vi "Relabel Annotation.vi"(0 "FSM.Graph In":refnum<class "FSM.Graph.lvclass">, 7 "Old Name":string, 9 "New Name":string) -> (4 "FSM.Graph Out":refnum<class "FSM.Graph.lvclass">)   [LabVIEW 2020, in "FSM.Graph.lvclass"]
uses:
  FSM.Graph.lvclass
  FSM.Graph.lvclass/FSM.Graph.ctl
  FSM.Edge/FSM.Edge.lvclass
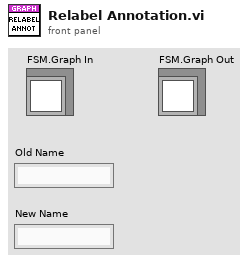
[diagram p1: front panel]
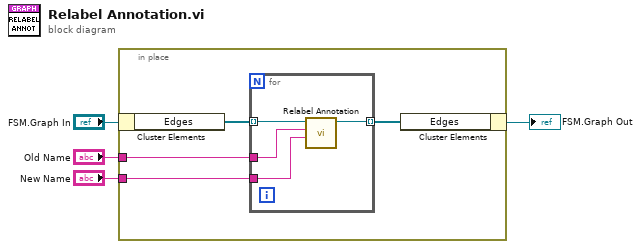
[diagram p0: block diagram]
diagram:
  n1 = in-place {
    in-place-border: "New Name" -> [w6]
    in-place-border: "Old Name" -> [w7]
    n2 = in-place-cluster #1("FSM.Graph In") -> ("Edges"=w8:refnum<class "FSM.Edge.lvclass">[])
    n3 = for {
      tunnel: w8 -> [w12] mode=indexing
      tunnel: w7 -> [w10]
      tunnel: w6 -> [w9]
      tunnel: [w11] -> w5 mode=indexing
      n4 = call "Relabel Annotation.vi"("New Name"=w9, "Old Name"=w10, "FSM.Edge in"=w12) -> ("FSM.Edge out"=w11:refnum<class "FSM.Edge.lvclass">)  [unwired: 7 in, 1 out]
    }
    n5 = in-place-cluster #1("Edges"=w5) -> (→"FSM.Graph Out":refnum<class "FSM.Graph.lvclass">)
  }
